vi "speichern.vi"(11 "VISA resource name":refnum<visa-resource-name>) -> ()   [LabVIEW 2019]
uses:
  Global 1.vi
panel:
  out "y":dbl
  out "x":dbl
  in  "stop":bool
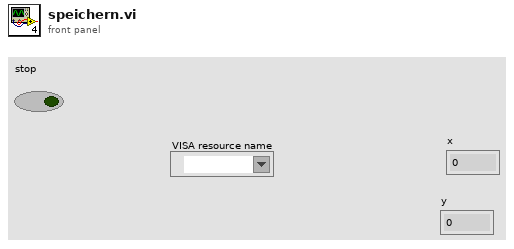
[diagram p1: front panel]
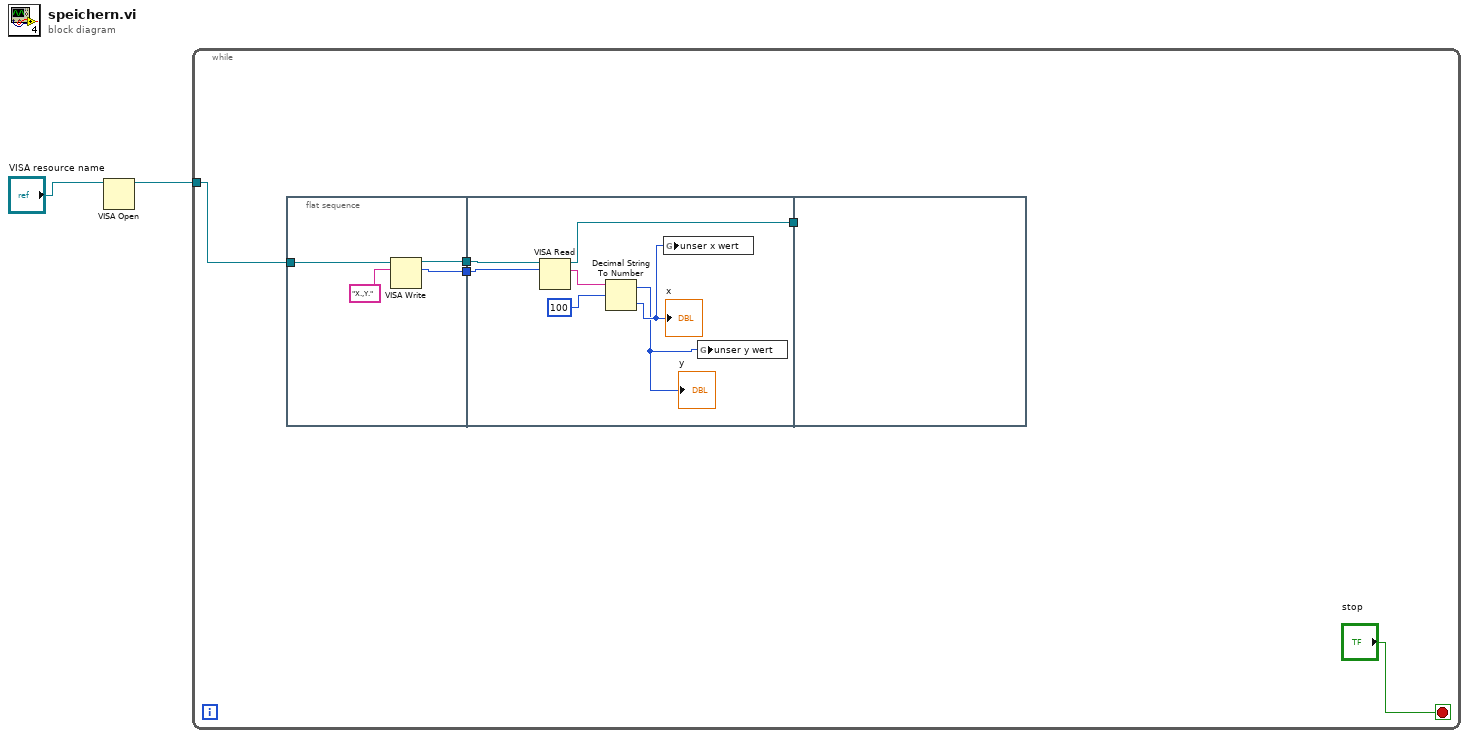
[diagram p0: block diagram]
diagram:
  n1 = VISA Open(VISA resource name="VISA resource name") -> (VISA resource name=w1:refnum<visa-resource-name>)  [unwired: 4 in, 1 out]
  n2 = while {
    tunnel: w1 -> [w6]
    stop <- "stop" stop-if-true
    n3 = flat-sequence {
      tunnel: w6 -> [w10]
      tunnel: [w9] -> w5
      tunnel: [w8] -> w4
      tunnel: w5 -> [w18]
      tunnel: w4 -> [w17]
      tunnel: [w14] -> w3
      tunnel: w3 -> [_]
      frame #0 {
        n4 = VISA Write(VISA resource name=w10, write buffer="X.,Y.") -> (VISA resource name out=w9:refnum<visa-resource-name>, return count=w8:u32)  [unwired: 1 in, 1 out]
      }
      frame #1 {
        n5 = VISA Read(VISA resource name=w18, byte count=w17) -> (VISA resource name out=w14:refnum<visa-resource-name>, read buffer=w16:string)  [unwired: 1 in, 2 out]
        n6 = Decimal String To Number(string=w16, offset=100) -> (offset past number=w12:i32, number=w15:i32)  [unwired: 1 in]
        "x" <- w15
        "y" <- w12
        n7 = global write "Global 1.vi" "unser x wert"(w15) -> ()
        n8 = global write "Global 1.vi" "unser y wert"(w12) -> ()
      }
      frame #2 {
      }
    }
  }
